vi "apply channel changes.vi"(8 "error in":errorcluster, 9 "new":refnum<class "Profibus channel.lvclass">, 10 "old":refnum<class "Profibus channel.lvclass">, 11 "Profibus Module configuration in":refnum<class "Profibus Module configuration.lvclass">) -> (0 "error out":errorcluster, 3 "Profibus Module configuration out":refnum<class "Profibus Module configuration.lvclass">)   [LabVIEW 2013, in "Profibus Module configuration.lvclass"]
uses:
  Profibus Module configuration.lvclass
  channel/Profibus channel.lvclass
  Profibus Module configuration.lvclass/Profibus Module configuration.ctl
  <vilib>/NI/Tag Bus/tag/tag descriptor.lvclass/tag descriptor.ctl
  <vilib>/NI/Tag Bus/tag/tag descriptor.lvclass
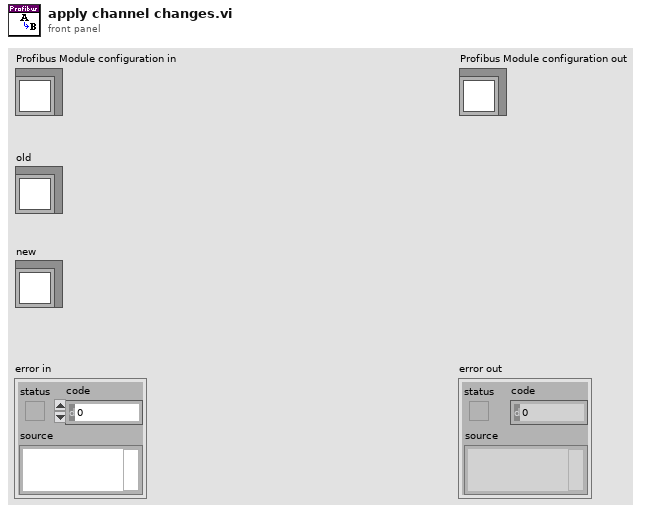
[diagram p1: front panel]
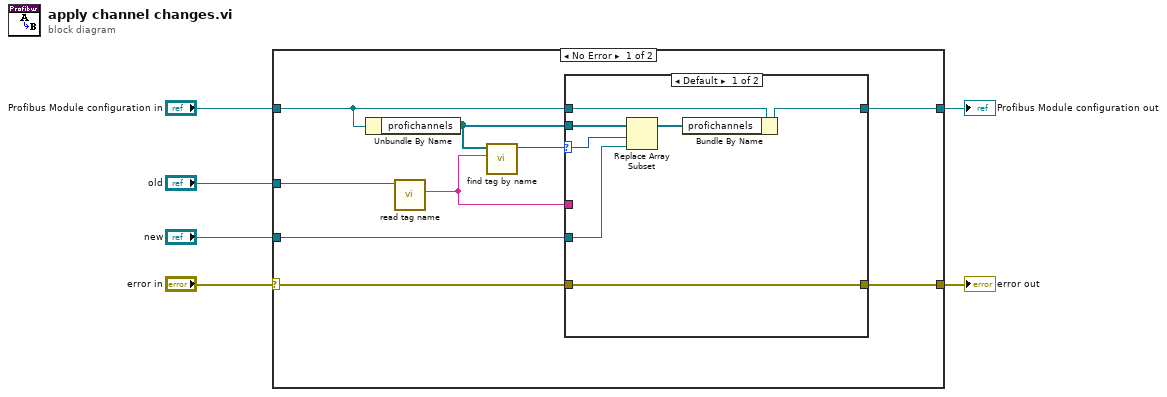
[diagram p0: block diagram]
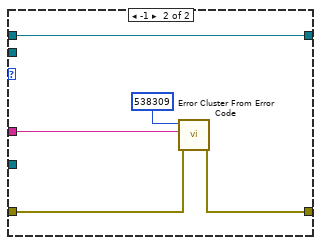
[diagram p2: hidden frame]
diagram:
  n1 = case shown="No Error" "error in" {
    selector: "error in" -> [w10 w29]
    tunnel: [w9 w29] -> w5
    tunnel: [w13 w28] -> w3
    tunnel: "Profibus Module configuration in" -> [w14 w28]
    tunnel: "old" -> [w15 _]
    tunnel: "new" -> [w11 _]
    frame No Error {
      n2 = Unbundle By Name(w14) -> ("profichannels"=w12:refnum<class "Profibus channel.lvclass">[])
      n3 = call <vilib>:"read tag name.vi"("system tag in"=w15) -> ("name"=w7:string)  [unwired: 8 in, 2 out]
      n4 = call <vilib>:"find tag by name.vi"("name"=w7, "tags in"=w12) -> ("index"=w8:i32)  [unwired: 9 in]
      n5 = case shown="Default" w8 {
        selector: w8 -> [w20 _]
        tunnel: w14 -> [w22 w27]
        tunnel: [w19 w27] -> w13
        tunnel: w12 -> [w21 _]
        tunnel: w11 -> [w17 _]
        tunnel: w7 -> [_ w25]
        tunnel: w10 -> [w16 w24]
        tunnel: [w16 w23] -> w9
        frame Default {
          n6 = Replace Array Subset(array=w21, new element=w17, index=w20) -> (w18:refnum<class "Profibus channel.lvclass">[])
          n7 = Bundle By Name(cluster=w22, "profichannels"=w18) -> (w19:refnum<class "Profibus Module configuration.lvclass">)
        }
        frame -1 {
          n8 = call <vilib>:"Error Cluster From Error Code.vi"("error in (no error)"=w24, "error message (\"\")"=w25, "error code (0)"=538309) -> ("error out"=w23:errorcluster)  [unwired: 6 in]
        }
      }
    }
    frame Error {
    }
  }
  "error out" <- w5
  "Profibus Module configuration out" <- w3
